vi "Create Hook from Template.vi"(8 "Error In":errorcluster, 9 "Call and Forget?":bool, 10 "Save Destination":path=path "", 11 "VI Template":refnum<vi>) -> (0 "Error Out":errorcluster)   [LabVIEW 2018, in "Tools Menu.lvlib"]
uses:
  Tools Menu.lvlib
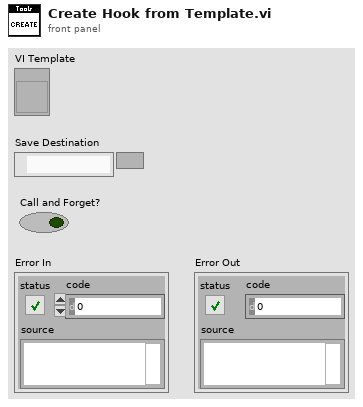
[diagram p1: front panel]
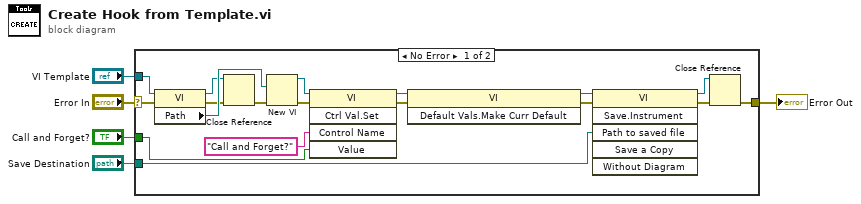
[diagram p0: block diagram]
diagram:
  n1 = case shown="No Error" "Error In" {
    selector: "Error In" -> [w6 w24]
    tunnel: "Save Destination" -> [w23 _]
    tunnel: [w22 w24] -> w4
    tunnel: "Call and Forget?" -> [w16 _]
    tunnel: "VI Template" -> [w9 _]
    frame No Error {
      n2 = property on="Property Node" class="VI"(reference=w9, error in=w6) -> (reference out=w8:refnum<vi>, error out=w7:errorcluster, "Path"=w11:path)
      n3 = Close Reference(reference=w8, error in (no error)=w7) -> (error out=w10:errorcluster)
      n4 = New VI(8:w10, 10:w11) -> (0:w15:errorcluster, 3:w12:refnum<vi>)  [unwired: 5 in]
      n5 = invoke class="VI" method="Ctrl Val.Set"(reference=w12, error in=w15, "Control Name"="Call and Forget?", "Value"=w16) -> (reference out=w17:refnum<vi>, error out=w19:errorcluster)  [unwired: 1 in, 3 out]
      n6 = invoke class="VI" method="Default Vals.Make Curr Default"(reference=w17, error in=w19) -> (reference out=w20:refnum<vi>, error out=w21:errorcluster)  [unwired: 1 in, 1 out]
      n7 = invoke class="VI" method="Save.Instrument"(reference=w20, error in=w21, "Path to saved file"=w23) -> (reference out=w13:refnum<vi>, error out=w14:errorcluster)  [unwired: 3 in, 4 out]
      n8 = Close Reference(reference=w13, error in (no error)=w14) -> (error out=w22:errorcluster)
    }
    frame Error {
    }
  }
  "Error Out" <- w4
